vi "simple DAQ.vi"() -> ()   [LabVIEW 2023]
uses:
  <vilib>/LabVIEW Targets/FPGA/cRIO/shared/nicrio_ModuleControls/nicrio_cRIO-9775_ContinuousDataRates4ChansRing.ctl
  <vilib>/LabVIEW Targets/FPGA/cRIO/shared/nicrio_ModuleControls/nicrio_BasicConversionTime.ctl
  <vilib>/rvi/Emulation/niFpgaGetClockAttributes.vi
  <vilib>/rvi/Emulation/niFpgaSctlEmulationGetInTimedLoop.vi
  <vilib>/rvi/Emulation/niFpgaEmulationReportErrorSimple.vi
  <vilib>/rvi/Emulation/niFpgaProcessEmulError.vi
  <vilib>/rvi/eio/common/nirviEmuTemplateMethod_errors.vi
  <vilib>/rvi/Emulation/niFpgaCriticalErrorInLSC.vi
  <vilib>/eio/EIONode/EIONode.xnode
panel:
  out "Stop":bool
  in  "Mod3/AO5":fxp<+/-,20,5>
  in  "Mod3/AO4":fxp<+/-,20,5>
  out "Mod1/AI3":fxp<+/-,17,5>
  out "Mod1/AI2":fxp<+/-,17,5>
  out "Mod1/AI1":fxp<+/-,17,5>
  out "Mod1/AI0":fxp<+/-,17,5>
  in  "Enable Low Pass Filter":T1={"Enable Low Pass Filter CH1"=TRUE, "Enable Low Pass Filter CH2"=TRUE, "Enable Low Pass Filter CH3"=TRUE, "Enable Low Pass Filter CH0"=TRUE}
  in  "Timing Mode":T2=enum."High Resolution"
  in  "Continuous Data Rate":T3=20 items=["1.000 MS/s (NI 9775)"=20, "833.333 KS/s (NI 9775)"=24, "714.286 KS/s (NI 9775)"=28, "625.000 KS/s (NI 9775)"=32, "555.556 KS/s (NI 9775)"=36, "500.000 KS/s (NI 9775)"=40, "454.545 KS/s (NI 9775)"=44, "416.667 KS/s (NI 9775)"=48, "384.615 KS/s (NI 9775)"=52, "357.143 KS/s (NI 9775)"=56, "333.333 KS/s (NI 9775)"=60, "312.500 KS/s (NI 9775)"=64, "294.118 KS/s (NI 9775)"=68, "277.778 KS/s (NI 9775)"=72, "263.158 KS/s (NI 9775)"=76, "250.000 KS/s (NI 9775)"=80, "238.095 KS/s (NI 9775)"=84, "227.273 KS/s (NI 9775)"=88, "217.391 KS/s (NI 9775)"=92, "208.333 KS/s (NI 9775)"=96, "200.000 KS/s (NI 9775)"=100, "192.308 KS/s (NI 9775)"=104, "185.185 KS/s (NI 9775)"=108, "178.571 KS/s (NI 9775)"=112, "172.414 KS/s (NI 9775)"=116, "166.667 KS/s (NI 9775)"=120, "161.290 KS/s (NI 9775)"=124, "156.250 KS/s (NI 9775)"=128, "151.515 KS/s (NI 9775)"=132, "147.059 KS/s (NI 9775)"=136, "142.857 KS/s (NI 9775)"=140, "138.889 KS/s (NI 9775)"=144, "135.135 KS/s (NI 9775)"=148, "131.579 KS/s (NI 9775)"=152, "128.205 KS/s (NI 9775)"=156, "125.000 KS/s (NI 9775)"=160, "121.951 KS/s (NI 9775)"=164, "119.048 KS/s (NI 9775)"=168, "116.279 KS/s (NI 9775)"=172, "113.636 KS/s (NI 9775)"=176, "111.111 KS/s (NI 9775)"=180, "108.696 KS/s (NI 9775)"=184, "106.383 KS/s (NI 9775)"=188, "104.167 KS/s (NI 9775)"=192, "102.041 KS/s (NI 9775)"=196, "100.000 KS/s (NI 9775)"=200, "50.000 KS/s (NI 9775)"=400, "33.333 KS/s (NI 9775)"=600, "25.000 KS/s (NI 9775)"=800, "20.000 KS/s (NI 9775)"=1000, "16.667 KS/s (NI 9775)"=1200, "14.286 KS/s (NI 9775)"=1400, "12.500 KS/s (NI 9775)"=1600, "11.111 KS/s (NI 9775)"=1800, "10.000 KS/s (NI 9775)"=2000, "9.091 KS/s (NI 9775)"=2200, "8.333 KS/s (NI 9775)"=2400, "7.692 KS/s (NI 9775)"=2600, "7.143 KS/s (NI 9775)"=2800, "6.667 KS/s (NI 9775)"=3000, "6.250 KS/s (NI 9775)"=3200, "5.882 KS/s (NI 9775)"=3400, "5.556 KS/s (NI 9775)"=3600, "5.000 KS/s (NI 9775)"=4000, "4.762 KS/s (NI 9775)"=4200, "4.545 KS/s (NI 9775)"=4400, "4.348 KS/s (NI 9775)"=4600, "4.167 KS/s (NI 9775)"=4800, "4.000 KS/s (NI 9775)"=5000, "3.846 KS/s (NI 9775)"=5200, "3.571 KS/s (NI 9775)"=5600, "3.333 KS/s (NI 9775)"=6000, "3.125 KS/s (NI 9775)"=6400, "2.941 KS/s (NI 9775)"=6800, "2.778 KS/s (NI 9775)"=7200, "2.632 KS/s (NI 9775)"=7600, "2.500 KS/s (NI 9775)"=8000, "2.381 KS/s (NI 9775)"=8400, "2.273 KS/s (NI 9775)"=8800, "2.174 KS/s (NI 9775)"=9200, "2.083 KS/s (NI 9775)"=9600, "2.000 KS/s (NI 9775)"=10000, "1.923 KS/s (NI 9775)"=10400, "1.852 KS/s (NI 9775)"=10800, "1.786 KS/s (NI 9775)"=11200, "1.724 KS/s (NI 9775)"=11600, "1.667 KS/s (NI 9775)"=12000, "1.613 KS/s (NI 9775)"=12400, "1.563 KS/s (NI 9775)"=12800, "1.515 KS/s (NI 9775)"=13200, "1.471 KS/s (NI 9775)"=13600, "1.429 KS/s (NI 9775)"=14000, "1.389 KS/s (NI 9775)"=14400, "1.351 KS/s (NI 9775)"=14800, "1.316 KS/s (NI 9775)"=15200, "1.282 KS/s (NI 9775)"=15600, "1.250 KS/s (NI 9775)"=16000, "1.220 KS/s (NI 9775)"=16400, "1.190 KS/s (NI 9775)"=16800, "1.163 KS/s (NI 9775)"=17200, "1.136 KS/s (NI 9775)"=17600, "1.111 KS/s (NI 9775)"=18000, "1.087 KS/s (NI 9775)"=18400, "1.064 KS/s (NI 9775)"=18800, "1.042 KS/s (NI 9775)"=19200, "1.020 KS/s (NI 9775)"=19600, "1.000 KS/s (NI 9775)"=20000, "0.980 KS/s (NI 9775)"=20400, "0.962 KS/s (NI 9775)"=20800, "0.943 KS/s (NI 9775)"=21200, "0.926 KS/s (NI 9775)"=21600, "0.909 KS/s (NI 9775)"=22000, "0.893 KS/s (NI 9775)"=22400, "0.877 KS/s (NI 9775)"=22800, "0.862 KS/s (NI 9775)"=23200, "0.847 KS/s (NI 9775)"=23600, "0.833 KS/s (NI 9775)"=24000, "0.820 KS/s (NI 9775)"=24400, "0.806 KS/s (NI 9775)"=24800, "0.794 KS/s (NI 9775)"=25200, "0.781 KS/s (NI 9775)"=25600, "0.694 KS/s (NI 9775)"=28800, "0.625 KS/s (NI 9775)"=32000, "0.568 KS/s (NI 9775)"=35200, "0.521 KS/s (NI 9775)"=38400, "0.446 KS/s (NI 9775)"=44800, "0.391 KS/s (NI 9775)"=51200, "0.347 KS/s (NI 9775)"=57600, "0.313 KS/s (NI 9775)"=64000]
  in  "Mod3/AO3":fxp<+/-,20,5>
  in  "Mod3/AO2":fxp<+/-,20,5>
  in  "Mod3/AO1":fxp<+/-,20,5>
  in  "Mod3/AO0":fxp<+/-,20,5>
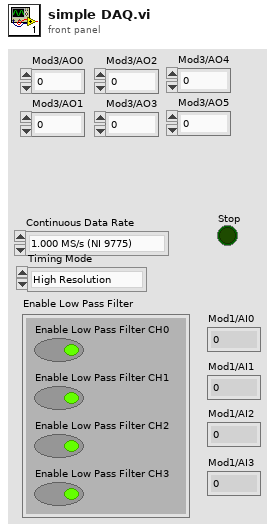
[diagram p1: front panel]
types:
  T1 = cluster{"Enable Low Pass Filter CH1":bool, "Enable Low Pass Filter CH2":bool, "Enable Low Pass Filter CH3":bool, "Enable Low Pass Filter CH0":bool}
  T2 = typedef "nicrio_BasicConversionTime.ctl" = enum8{"High Speed", "High Resolution"}
  T3 = typedef "nicrio_cRIO-9775_ContinuousDataRates4ChansRing.ctl" = u16
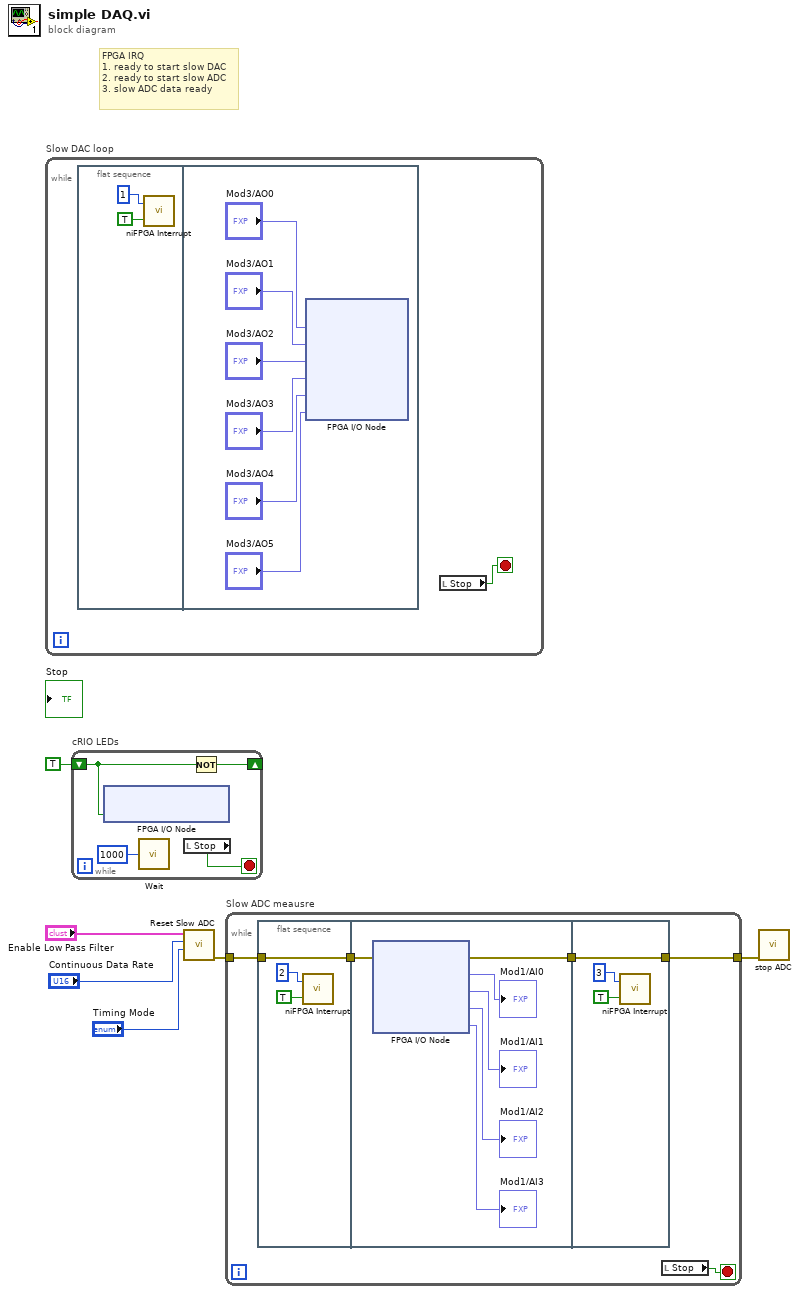
[diagram p0: block diagram]
diagram:
  # "FPGA IRQ\n1. ready to start slow DAC\n2. ready to start slow ADC\n3. slow ADC data ready"
  n1 = while "Slow DAC loop" {
    stop <- w7 stop-if-true
    n2 = flat-sequence {
      frame #0 {
        n3 = call <vilib>:"niFPGA Interrupt.vi"("Wait Until Cleared (F)"=TRUE, "IRQ Number (0)"=u8 1) -> ()  [unwired: 1 in]
      }
      frame #1 {
        n4 = xnode "FPGA I/O Node"("Mod3/AO0"="Mod3/AO0", "Mod3/AO1"="Mod3/AO1", "Mod3/AO2"="Mod3/AO2", "Mod3/AO3"="Mod3/AO3", "Mod3/AO4"="Mod3/AO4", "Mod3/AO5"="Mod3/AO5") -> ()  [unwired: 6 in, 6 out]
      }
    }
    n5 = local read "Stop"() -> (w7:bool)
  }
  n6 = while "cRIO LEDs" {
    shift-right: [w17] -> _
    shift-left: TRUE ("USER FPGA LED") -> [w18]
    stop <- w16 stop-if-true
    n7 = xnode "FPGA I/O Node"("USER FPGA LED"=w18) -> ()  [unwired: 1 in, 1 out]
    n8 = call "Wait"("Count(mSec)"=u32 1000) -> ()  [unwired: 1 out]
    n9 = local read "Stop"() -> (w16:bool)
    n10 = Not(x=w18) -> (.not. x?=w17:bool)
  }
  n11 = call "Reset Slow ADC.vi"("Timing Mode"="Timing Mode", "Continuous Data Rate"="Continuous Data Rate", "Enable Low Pass Filter"="Enable Low Pass Filter") -> ("error out"=w4:errorcluster)  [unwired: 8 in]
  n12 = while "Slow ADC meausre" {
    tunnel: w4 -> [w23]
    tunnel: [w22] -> w5
    stop <- w20 stop-if-true
    n13 = flat-sequence {
      tunnel: [w25] -> w24
      tunnel: w23 -> [w25]
      tunnel: w24 -> [w29]
      tunnel: [w28] -> w21
      tunnel: [w34] -> w22
      tunnel: w21 -> [w34]
      frame #0 {
        n14 = call <vilib>:"niFPGA Interrupt.vi"("Wait Until Cleared (F)"=TRUE, "IRQ Number (0)"=u8 2) -> ()  [unwired: 1 in]
      }
      frame #1 {
        n15 = xnode "FPGA I/O Node"("error in"=w29) -> ("error out"=w28:errorcluster, "Mod1/AI0"=→"Mod1/AI0":fxp<+/-,17,5>, "Mod1/AI1"=→"Mod1/AI1":fxp<+/-,17,5>, "Mod1/AI2"=→"Mod1/AI2":fxp<+/-,17,5>, "Mod1/AI3"=→"Mod1/AI3":fxp<+/-,17,5>)  [unwired: 4 in, 4 out]
      }
      frame #2 {
        n16 = call <vilib>:"niFPGA Interrupt.vi"("Wait Until Cleared (F)"=TRUE, "IRQ Number (0)"=u8 3) -> ()  [unwired: 1 in]
      }
    }
    n17 = local read "Stop"() -> (w20:bool)
  }
  n18 = call "stop ADC.vi"("error in"=w5) -> ()  [unwired: 10 in, 1 out]
